vi "ge_CalibrateSingleChan.vi"(5 "Chassis Name":string, 6 "Ctrl Name":string, 7 "MeasType":T4=enum."Dynamic", 8 "error in":errorcluster, 9 "Row":i32, 10 "ItemNames":string[](array[string]), 11 "ge_DAQManDefinitions":T1) -> (0 "error out":errorcluster, 2 "Cell Contents":T2[](array[typedef]))   [LabVIEW 2018]
uses:
  Custom Ctrls/ge_MeasType.ctl
  Custom Ctls Table/ge_CellContents.ctl
  <vilib>/Utility/miscctls.llb/LVPoint32TypeDef.ctl
  Common/Controls/DAQMan Definitions.ctl
  Classes/Measurements/Class Channel/Channel.lvclass
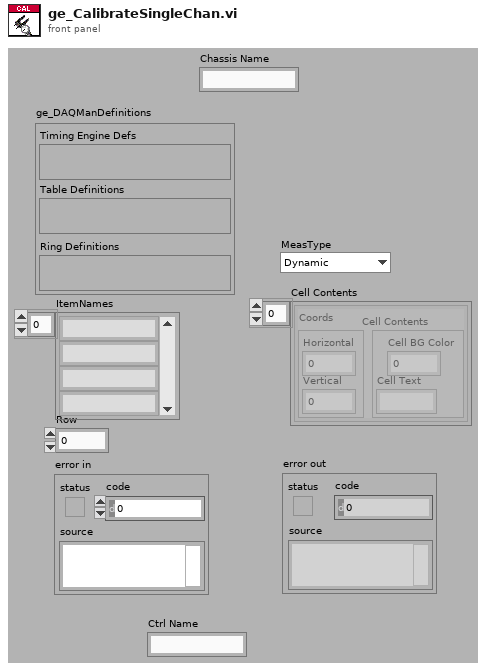
[diagram p1: front panel]
types:
  T1 = typedef "DAQMan Definitions.ctl" = cluster{"Timing Engine Defs":variant, "Table Definitions":variant, "Ring Definitions":variant}
  T2 = typedef "ge_CellContents.ctl" = cluster{"Cell Contents":cluster{"Cell Text":string, "Cell BG Color":u32}, "Coords":T3}
  T3 = typedef "LVPoint32TypeDef.ctl" = cluster{"Horizontal":i32, "Vertical":i32}
  T4 = typedef "ge_MeasType.ctl" = enum16{"Voltage", "Frequency", "Tachometer", "Dynamic", "Thermocouple", "RTD", "Strain", "Current", "Resistance"}
  T5 = typedef "HeaderNames.ctl" = enum16{"Channel", "Device", "Spacer", "Description", "MB", "Range", "Terminal", "Coupling", "Thresh (V)", "Pulse/Rev", "Slope", "Min EU", "Min RPM", "mV/EU", "Iex", "Temp Units", "Type", "CJC Src", "CJC Val", "Ro", "Wire Cfg", "Strain Mode", "Vex", "Bridge Type", "GF", "Gauge Res", "Poisson", "Lead Res", "Init Strain", "GAF", "Scale", "Offset", "Unit (EU)", "dB?", "dB Ref", "Cal Mag", "Cal Units", "Max Temp", "Min Temp", "Max Strain", "Min Strain"}
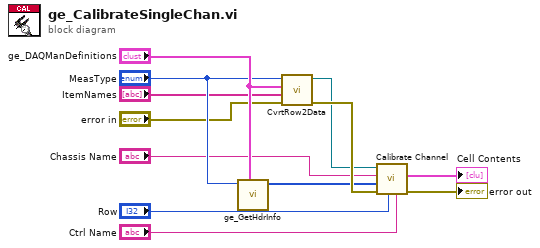
[diagram p0: block diagram]
diagram:
  n1 = call "ge_GetHdrInfo.vi"("ge_DAQManDefinitions"="ge_DAQManDefinitions", "MeasType"="MeasType") -> ("Hdr Name"=w4:T5[])  [unwired: 7 in, 2 out]
  n2 = call "CvrtRow2Data.vi"("error in (no error)"="error in", "Item Names"="ItemNames", "ge_DAQManDefinitions"="ge_DAQManDefinitions", "MeasType"="MeasType") -> ("error out"=w8:errorcluster, "Channel out"=w7:refnum<class "Channel.lvclass">)  [unwired: 6 in]
  n3 = call-dynamic "Calibrate Channel.vi"("Ctrl Name"="Ctrl Name", "Row"="Row", "error in (no error)"=w8, "Hdr Names"=w4, "Chassis Name"="Chassis Name", "Channel in"=w7) -> ("error out"=→"error out":errorcluster, "Cell Contents"=→"Cell Contents":T2[])  [unwired: 4 in]
